vi "Get Object Parameter - Null.vi"(0 "JSON Tree In (JSON Object)":variant, 5 "Parameter Name":string, 11 "error in (no error)":errorcluster) -> (4 "JSON Tree Out Passthrough":variant, 6 "JSON Null Value":variant, 10 "is JSON Null?":bool, 15 "error out":errorcluster)   [LabVIEW 2015, in "i3-json.lvlib"]
doc: "Use this template to build a VI to use as a subVI."
uses:
  i3-json.lvlib
  JSON Types/JSON Type.ctl
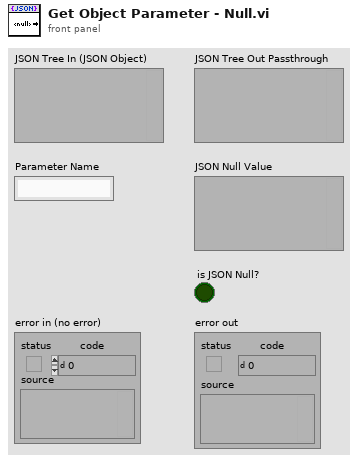
[diagram p1: front panel]
types:
  T1 = typedef "i3-json.lvlib/JSON Type.ctl" = enum8{"JSON Compatible", "JSON Array", "JSON Object", "JSON Null", "Double", "String", "Boolean", "Unknown"}
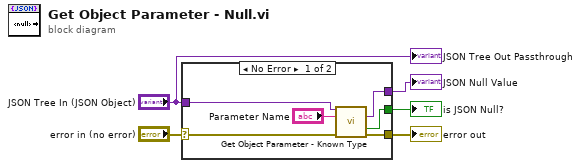
[diagram p0: block diagram]
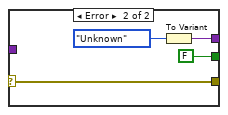
[diagram p2: hidden frame]
diagram:
  n1 = case shown="No Error" "error in (no error)" {
    selector: "error in (no error)" -> [w10 w15]
    tunnel: [w9 w15] -> w4
    tunnel: "JSON Tree In (JSON Object)" -> [w11 _]
    tunnel: [w8 FALSE ("is JSON Null?")] -> w3
    tunnel: [w7 w14] -> w2
    frame No Error {
      n2 = call "Get Object Parameter - Known Type.vi"("JSON Tree In (JSON Object)"=w11, "Parameter Name"="Parameter Name", "error in (no error)"=w10) -> ("Value"=w7:variant, "is JSON Null?"=w8:bool, "error out"=w9:errorcluster)  [unwired: 7 in, 3 out]
    }
    frame Error {
      n3 = To Variant(anything=JSON_Type."Unknown" ("JSON Type")) -> (Variant=w14:variant)
    }
  }
  "error out" <- w4
  "is JSON Null?" <- w3
  "JSON Null Value" <- w2
  "JSON Tree Out Passthrough" <- "JSON Tree In (JSON Object)"
